vi "LWConexPSD_Disconnect.vi"(2 "error in (no error)":errorcluster caption="error in", 3 "Component ID":i32, 4 "ConexPSD Référence":refnum<k24>) -> (0 "Error out":errorcluster caption="error out")   [LabVIEW 2010]
uses:
  D:/LabVIEW_program/노트북LabVIEW/THz Time/THz Time(SR830_ESP300_SHOT202_TEC or Nova_PSD)_PulseE_LGS/Dll/Newport.CONEXPSD.CommandInterface.DLL
  Dll/Newport.CONEXPSD.CommandInterface.DLL
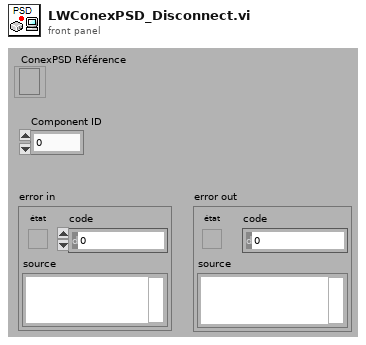
[diagram p1: front panel]
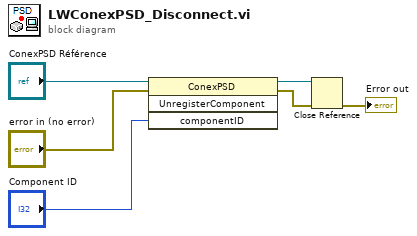
[diagram p0: block diagram]
diagram:
  n1 = invoke class="ConexPSD" method="UnregisterComponent"(reference="ConexPSD Référence", error in="error in (no error)", "componentID"="Component ID") -> (reference out=w6:refnum<k24>, error out=w5:errorcluster)  [unwired: 1 in, 2 out]
  n2 = Close Reference(reference=w6, error in (no error)=w5) -> (error out=→"Error out":errorcluster)
